vi "Set Bold Text.vi"(1 "prefix adjustment":i32, 3 "error in":errorcluster, 4 "Length":i32[](array[numeric]), 5 "Start":i32[](array[numeric]), 6 "text":refnum<vi>) -> (0 "error out":errorcluster)   [LabVIEW 2010]
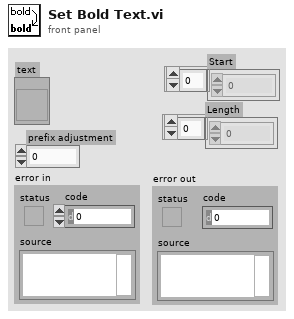
[diagram p1: front panel]
types:
  T1 = cluster{"Selection Start":u32, "Selection End":u32}
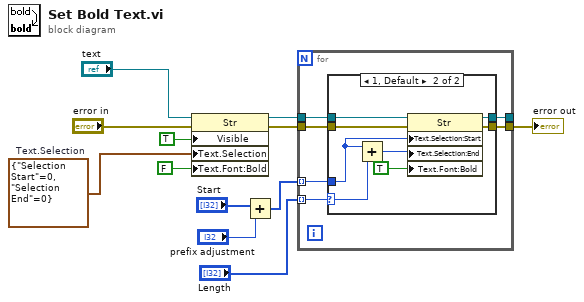
[diagram p0: block diagram]
diagram:
  w10 = T1 {"Selection Start"=0, "Selection End"=0}  # Text.Selection
  n1 = property on="Property Node" class="Str"(reference="text", error in="error in", "Visible"=TRUE, "Text.Selection"=w10, "Text.Font:Bold"=FALSE) -> (reference out=w8:refnum<vi>, error out=w9:errorcluster)
  n2 = Add(x="Start", y="prefix adjustment") -> (x+y=w3:i32[])
  n3 = for {
    tunnel: w8 -> [w18]
    tunnel: w9 -> [w17]
    tunnel: [w16] -> w5
    tunnel: w3 -> [w15] mode=indexing
    tunnel: "Length" -> [w13] mode=indexing
    tunnel: [w14] -> _
    n4 = case shown="1, Default" w13 {
      selector: w13 -> [_ w21]
      tunnel: w18 -> [w20 w28]
      tunnel: w17 -> [w19 w27]
      tunnel: [w19 w24] -> w16
      tunnel: w15 -> [_ w23]
      tunnel: [w20 w22] -> w14
      frame 0 {
      }
      frame 1, Default {
        n5 = Add(x=w23, y=w21) -> (x+y=w26:i32)
        n6 = property on="Property Node" class="Str"(reference=w28, error in=w27, "Text.Selection:Start"=w23, "Text.Selection:End"=w26, "Text.Font:Bold"=TRUE) -> (reference out=w22:refnum<vi>, error out=w24:errorcluster)
      }
    }
  }
  "error out" <- w5
